vi "HEWH RLT Selected MW100 TCs.vi"(4 "Collect Power Data":bool, 5 "Show Flow Data":bool, 6 "Station ID":string="A", 7 "Current Drawing Station":string="A", 8 "Error In":errorcluster, 9 "Station A Channels, MW100":string[][](array[string])=[["T1 - IN", "11"], ["T1 - OUT", "13"]], 10 "MW100 Full Data":string[][](array[string])=[["Voltage (V)", "0.000"], ["RMS Current (Amps)", "0.000"], ["Power (Watts)", "0.000"], ["Watt Hours (Wh)", "0.000"], ["Voltage Total Harmonic Distortion", "0.000"], ["Frequency (Hz)", "0.000"], ["Apparent Power (VA)", "0.000"], ["Power Factor", "0.000"], ["Current Crest Factor", "0.000"], ["Voltage Crest Factor", "0.000"], ["Integration Time (sec)", "0.000"], ["Intellifaucet Valve % Open", "0.000"], ["Draw Count", "1"], ["T1", "10.2"], ["T2", "20"], ["T3", "0.000"], ["T4", "0.000"], ["T5", "0.000"], ["T6", "0.000"], ["T7", "0.000"], ["T8", "0.000"], ["T9", "0.000"], ["T10", "0.000"], ["TC Tree Average", "0.000"], ["TC Down", "0.000"], ["RTD IN", "0.000"], ["RTD Out", "0.000"], ["RTD Ambient", "0.000"], ["Totalized Flow (Linear Link) - Calculated (Gallons)", "0.000"], ["Flow Rate (Linear Link) - Calculated (GPM)", "0.000"], ["Pressure - HI1", "0.000"], ["Pressure - HI2", "0.000"], ["Pressure - LOW", "0.000"], ["Pressure - PIN", "0.000"]], 11 "LV Program":T1=enum."HEWH") -> (0 "Error Out":errorcluster, 1 "TC Data":string[][](array[string]), 2 "RMS Current (Amps)":dbl, 3 "Data (Label,Data)":string[][](array[string])=[["Voltage (V)", "0.000"], ["RMS Current (Amps)", "0.000"], ["Power (Watts)", "0.000"], ["Watt Hours (Wh)", "0.000"], ["Voltage Total Harmonic Distortion", "0.000"], ["Frequency (Hz)", "0.000"], ["Apparent Power (VA)", "0.000"], ["Power Factor", "0.000"], ["Current Crest Factor", "0.000"], ["Voltage Crest Factor", "0.000"], ["Integration Time (sec)", "0.000"], ["Intellifaucet Valve % Open", "0.000"], ["TC Tree Average", "0.000"], ["TC Down", "0.000"], ["RTD IN", "0.000"], ["RTD Out", "0.000"], ["RTD Ambient", "0.000"], ["Totalized Flow (Linear Link) - Calculated (Gallons)", "0.000"], ["Flow Rate (Linear Link) - Calculated (GPM)", "0.000"], ["Pressure - HI1", "0.000"], ["Pressure - HI2", "0.000"], ["Pressure - LOW", "0.000"], ["Pressure - PIN", "0.000"]])   [LabVIEW 2016]
uses:
  Utility/Save File/File Setup (Public)/Type Definition/Save File DOE LabView Program.ctl
  Type Definitions/PRAT Channel Settings.ctl
  Custom Instrument Control/MW100/Type Definitions/HEWH MW100 Channel Numbers.ctl
  Utility/Save File/File Setup.lvlib
panel:
  out "All Other Data (NO TC's)":string[][](array[string])
  in  "PRAT Example Data":string[][](array[string])=[["Power (Watts) - Station A", "1"], ["Power (Watts) - Station B", "2"], ["Power (Watts) - Station C", "3"], ["Power (Watts) - Station D", "4"], ["WattHours (Wh) - Station A", "1"], ["WattHours (Wh) - Station B", "2"], ["WattHours (Wh) - Station C", "3"], ["WattHours (Wh) - Station D", "4"], ["T1", "1"], ["T2", "2"], ["T3", "3"], ["T4", "4"], ["Ambient Temperature", "100"], ["Extra Temperature", "200"], ["Draw Count", "1"], ["Program Status", "Testing B..."]]
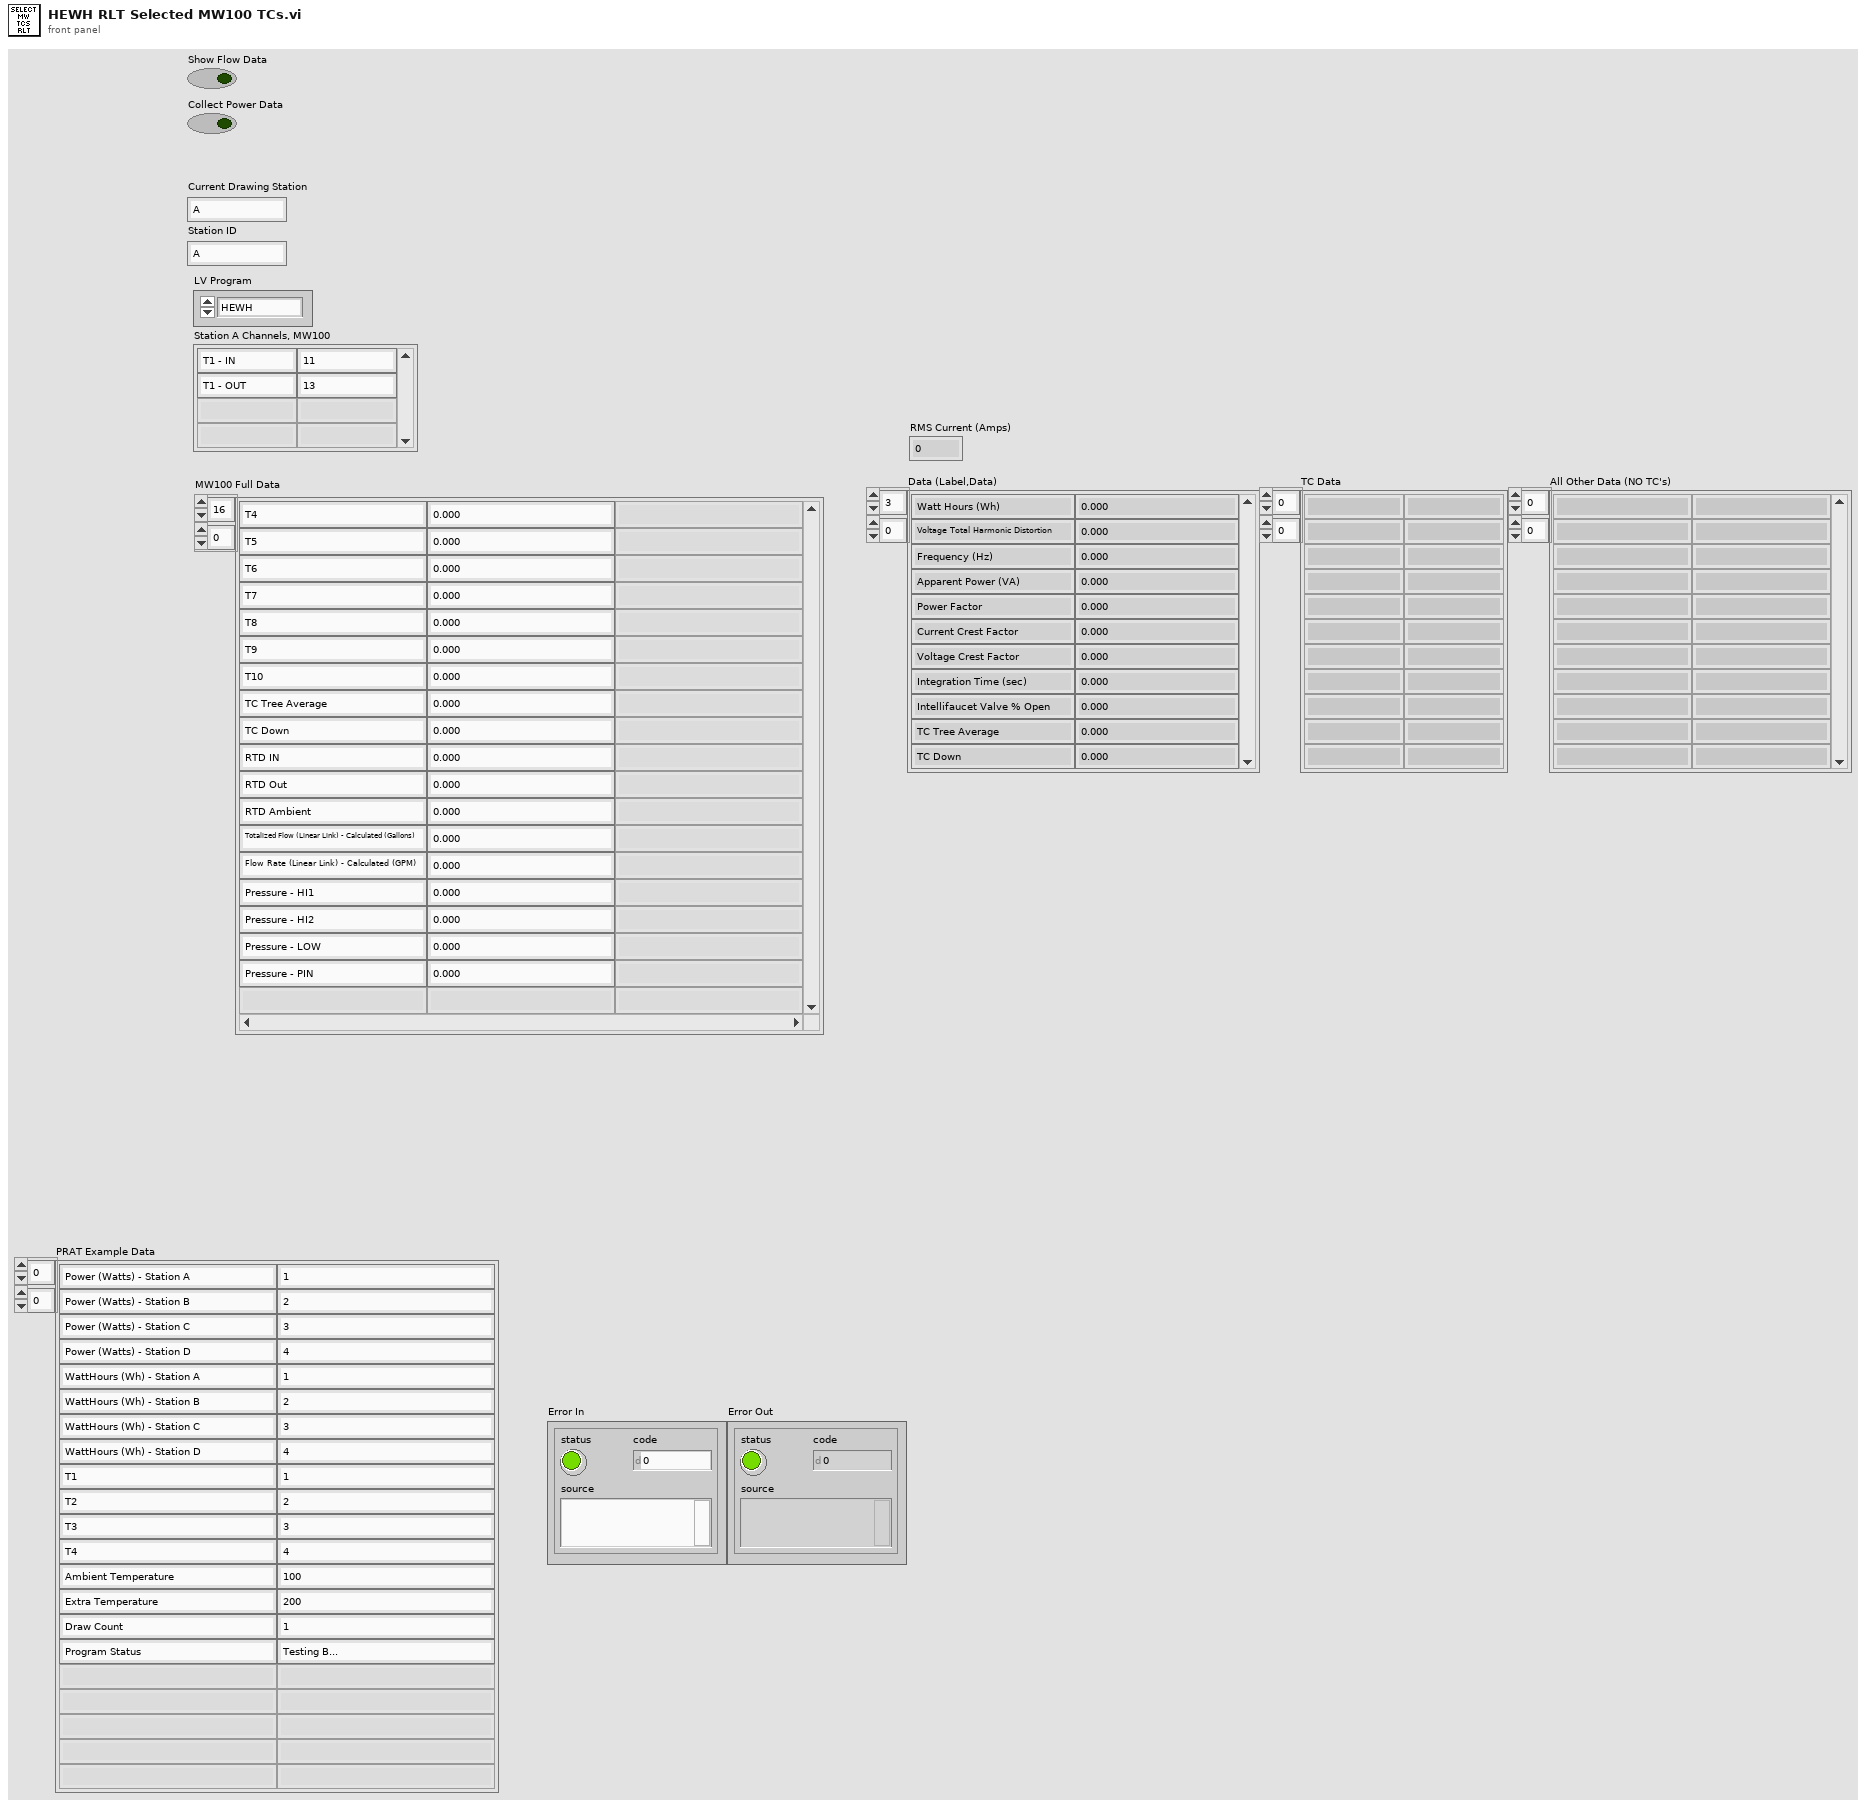
[diagram p1: front panel]
types:
  T1 = typedef "File Setup.lvlib/Save File DOE LabView Program.ctl" = enum16{"No Name Found", "DOE Stand", "Dishwasher Kitchen", "Portable Stand", "HEWH", "Dryer", "Dryer WILT", "HCC", "PRAT", "HEWH RLT", "Refrigeration"}
  T2 = typedef "PRAT Channel Settings.ctl" = string
  T3 = typedef "HEWH MW100 Channel Numbers.ctl" = string
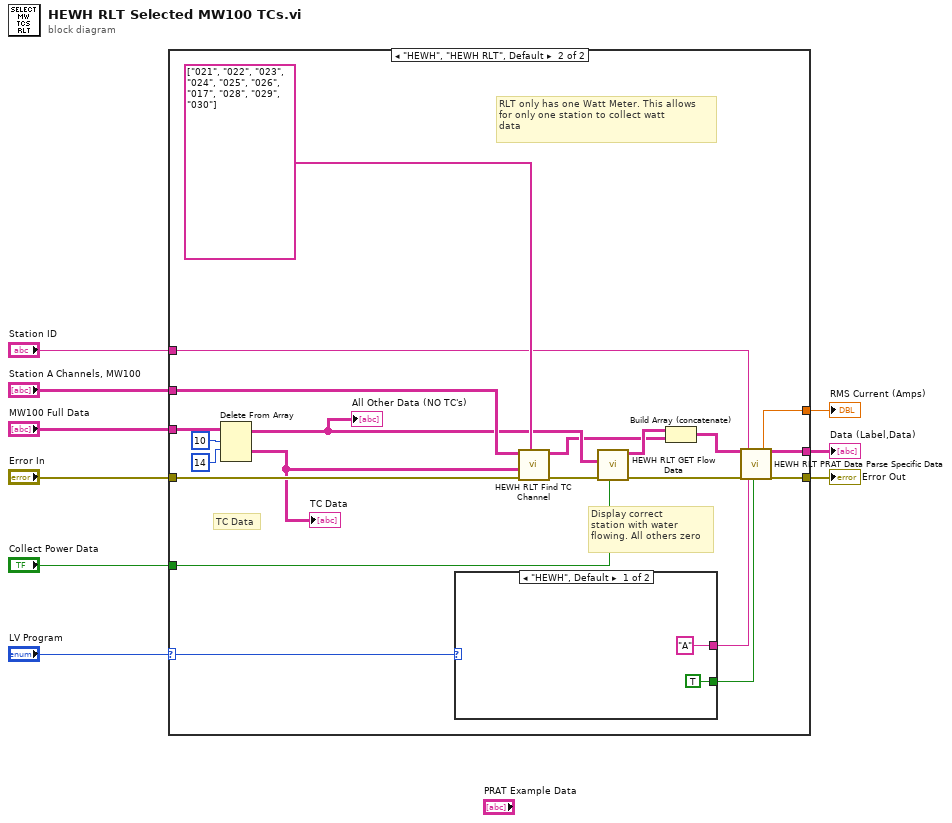
[diagram p0: block diagram]
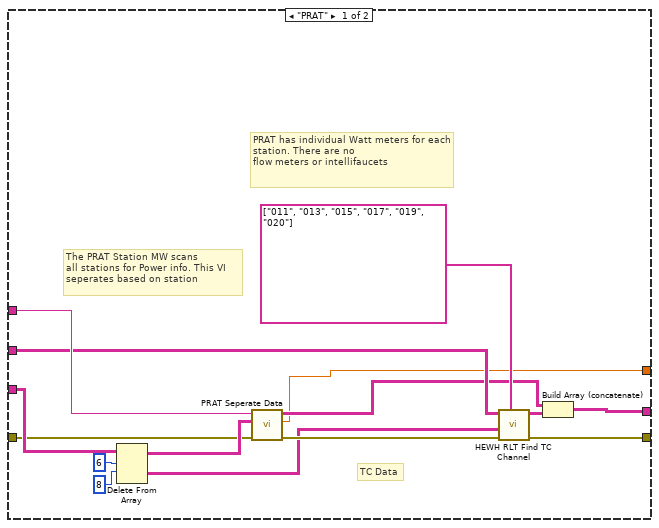
[diagram p2: hidden frame]
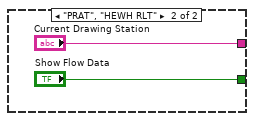
[diagram p3: hidden frame]
diagram:
  n1 = case shown="\"HEWH\", \"HEWH RLT\", Default" "LV Program" {
    selector: "LV Program" -> [_ w27]
    tunnel: "MW100 Full Data" -> [w22 w45]
    tunnel: "Station A Channels, MW100" -> [w14 w36]
    tunnel: [w11 w40] -> w9
    tunnel: "Error In" -> [w18 w41]
    tunnel: [w23 w39] -> w6
    tunnel: "Station ID" -> [w16 w38]
    tunnel: "Collect Power Data" -> [_ w29]
    tunnel: [w10 w26] -> w1
    frame "PRAT" {
      # "PRAT has individual Watt meters for each station. There are no\nflow meters or intellifaucets"
      # "The PRAT Station MW scans\nall stations for Power info. This VI\nseperates based on station"
      # "TC Data"
      n2 = Delete From Array(array=w22, length=6 ("index (row)"), index (row)=8) -> (deleted portion=w15:string[][], array with subset deleted=w20:string[][])  [unwired: 1 in]
      n3 = call "PRAT Seperate Data.vi"("Error In"=w18, "PRAT Power Data"=w20, "Prat Station"=w16) -> ("Error Out"=w17:errorcluster, "RMS Current (Amps)"=w10:dbl, "Station Power Data"=w13:string[][])  [unwired: 6 in]
      n4 = call "HEWH RLT Find TC Channel.vi"("Program Channel Locations In"=T2[] ["011", "013", "015", "017", "019", "020"], "Error In"=w17, "TC Data"=w15, "Station A Channels, MW100"=w14) -> ("Error Out"=w23:errorcluster, "TC Data"=w12:string[][])  [unwired: 6 in]
      n5 = Build Array (concatenate)(w13, w12) -> (w11:string[][])
    }
    frame "HEWH", "HEWH RLT", Default {
      # "Display correct\nstation with water\nflowing. All others zero"
      # "RLT only has one Watt Meter. This allows\nfor only one station to collect watt \ndata"
      # "TC Data"
      n6 = Delete From Array(array=w45, length=10, index (row)=14 ("disabled index (row)")) -> (deleted portion=w37:string[][], array with subset deleted=w35:string[][])  [unwired: 1 in]
      "TC Data" <- w37
      "All Other Data (NO TC's)" <- w35
      n7 = case shown="\"HEWH\", Default" w27 {
        tunnel: ["A" ("Current Drawing Station") "Current Drawing Station"] -> w28
        tunnel: [TRUE ("Show Flow Data") "Show Flow Data"] -> w25
        frame "HEWH", Default {
        }
        frame "PRAT", "HEWH RLT" {
        }
      }
      n8 = call "HEWH RLT Find TC Channel.vi"("Program Channel Locations In"=T3[] ["021", "022", "023", "024", "025", "026", "017", "028", "029", "030"] ("Array"), "Error In"=w41, "TC Data"=w37, "Station A Channels, MW100"=w36) -> ("Error Out"=w34:errorcluster, "TC Data"=w32:string[][])  [unwired: 6 in]
      n9 = call "HEWH RLT GET Flow Data.vi"("Collect Power Data"=w29, "Error In"=w34, "All Other Data (NO TC's) in"=w35) -> ("Error Out"=w30:errorcluster, "All Other Data (NO TC's) out"=w33:string[][])  [unwired: 7 in]
      n10 = Build Array (concatenate)(w33, w32) -> (w31:string[][])
      n11 = call "HEWH RLT PRAT Data Parse Specific Data.vi"("Data (Label,Data) In"=w31, "Error In"=w30, "Station ID"=w38, "Current Drawing Station"=w28, "Show Flow Data"=w25) -> ("Current (Amps)"=w26:dbl, "Data (Label,Data) Out"=w40:string[][], "Error Out"=w39:errorcluster)  [unwired: 12 in]
    }
  }
  "Data (Label,Data)" <- w9
  "Error Out" <- w6
  "RMS Current (Amps)" <- w1
